vi "02-StateMachineWithEvStr.vi"() -> ()   [LabVIEW 2017]
uses:
  Support/01-Typedef.ctl
panel:
  in  "Msg Button":bool
  in  "stop":bool
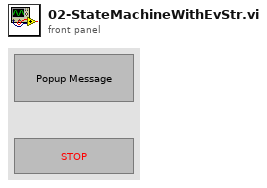
[diagram p1: front panel]
types:
  T1 = typedef "01-Typedef.ctl" = enum16{"Init", "Button", "Idle", "Exit"}
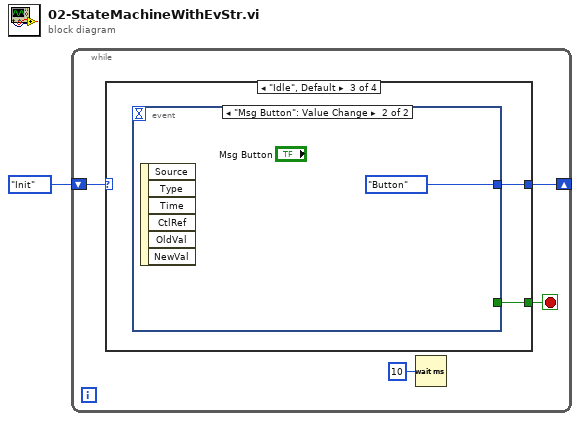
[diagram p0: block diagram]
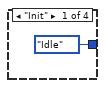
[diagram p2: hidden frame]
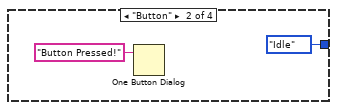
[diagram p3: hidden frame]
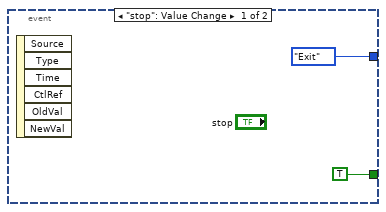
[diagram p4: hidden frame]
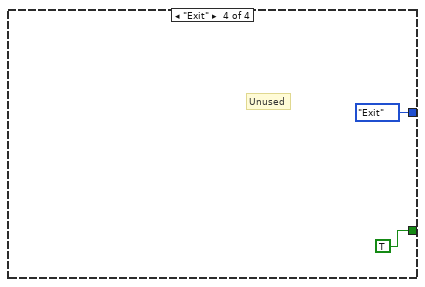
[diagram p5: hidden frame]
diagram:
  n1 = while {
    shift-right: [w2] -> _
    shift-left: 01-Typedef."Init" ("Enum") -> [w5]
    stop <- w4 stop-if-true
    n2 = case shown="\"Idle\", Default" w5 {
      tunnel: [_ _ w10 TRUE] -> w4
      tunnel: [01-Typedef."Idle" ("Enum") 01-Typedef."Idle" ("Enum") w9 01-Typedef."Exit" ("Enum")] -> w2
      frame "Init" {
      }
      frame "Button" {
        n3 = One Button Dialog(message="Button Pressed!") -> ()  [unwired: 1 in, 1 out]
      }
      frame "Idle", Default {
        n4 = event shown="[1] \"Msg Button\": Value Change" {
          selector: _ -> [_ _]
          dyn-events: _ -> [_ _]
          timeout: _ -> [_ _]
          tunnel: [TRUE _] -> w10
          tunnel: [01-Typedef."Exit" ("t") 01-Typedef."Button" ("Enum")] -> w9
          event "stop": Value Change {
            n5 = event-data() -> ()  [unwired: 1 in, 6 out]
          }
          event "Msg Button": Value Change {
            n6 = event-data() -> ()  [unwired: 1 in, 6 out]
          }
        }
      }
      frame "Exit" {
        # "Unused"
      }
    }
    n7 = Wait (ms)(milliseconds to wait=u32 10) -> ()  [unwired: 1 out]
  }
